vi "CTRE_Phoenix_CANdle_GetFaults.vi"(8 "error in":errorcluster, 11 "CTRE_CANdle_DeviceRef":T2) -> (0 "error out":errorcluster, 2 "Faults":T1, 3 "CTRE_CANdle_DeviceRef":T2)   [LabVIEW 2020]
doc: "Gets the current fault status of the CANdle."
uses:
  <vilib>/Rock Robotics/WPI/ThirdParty/Phoenix-LabVIEW/CANdle/Controls/CTRE_Phoenix_CANdle_DeviceRef.ctl
  <vilib>/Rock Robotics/WPI/ThirdParty/Phoenix-LabVIEW/CANdle/Controls/CTRE_Phoenix_CANdle_Faults.ctl
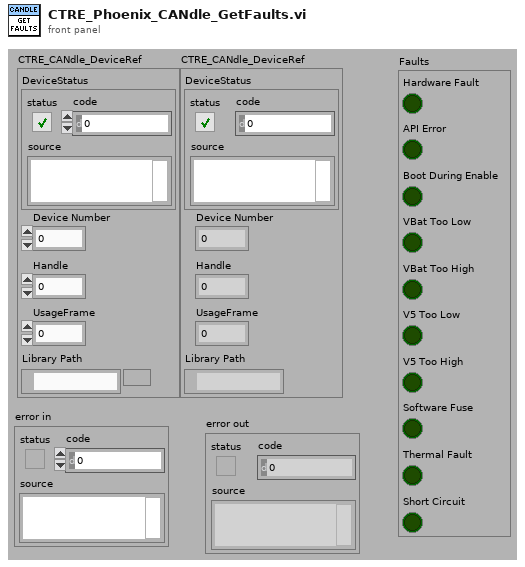
[diagram p1: front panel]
types:
  T1 = typedef "CTRE_Phoenix_CANdle_Faults.ctl" = cluster{"Hardware Fault":bool, "API Error":bool, "Boot During Enable":bool, "VBat Too Low":bool, "VBat Too High":bool, "V5 Too Low":bool, "V5 Too High":bool, "Software Fuse":bool, "Thermal Fault":bool, "Short Circuit":bool}
  T2 = typedef "CTRE_Phoenix_CANdle_DeviceRef.ctl" = cluster{"DeviceStatus":errorcluster, "Device Number":u8, "Handle":u64, "UsageFrame":u32, "Library Path":path}
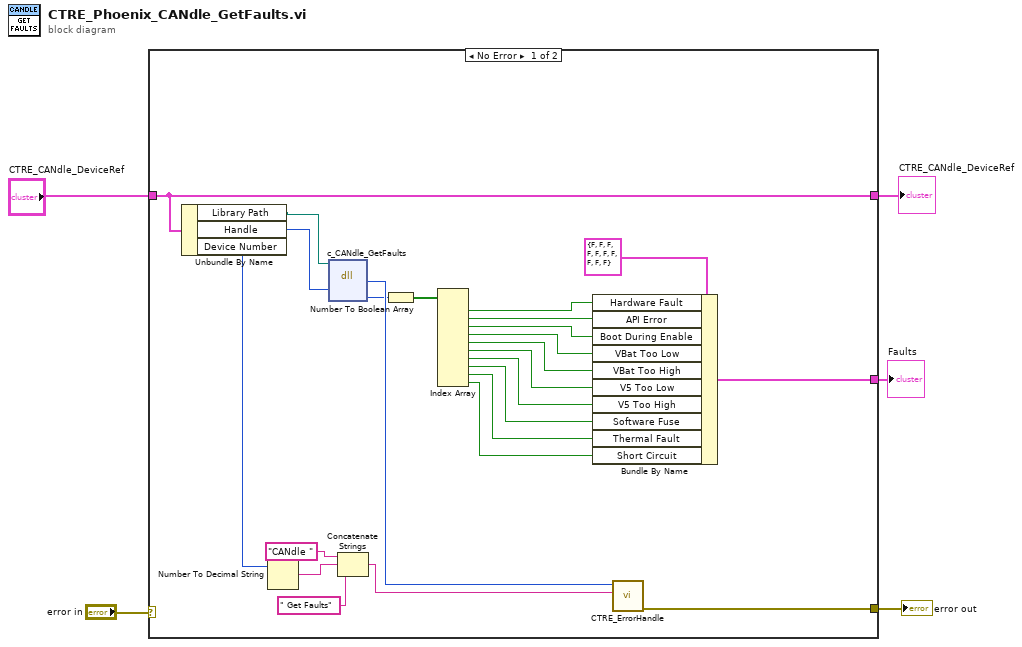
[diagram p0: block diagram]
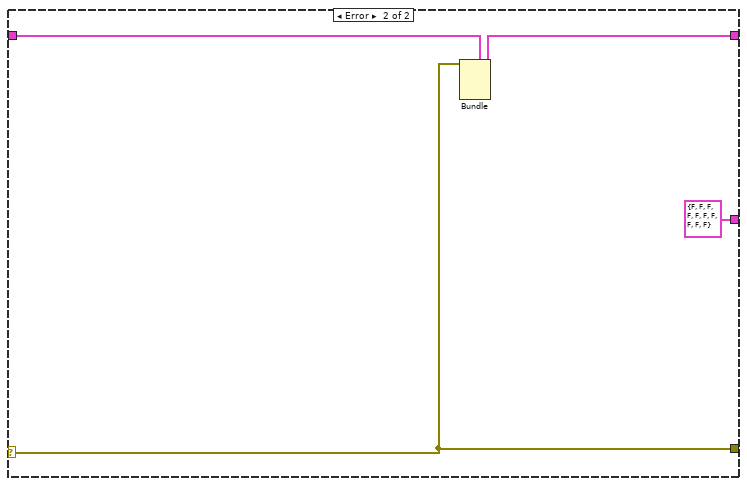
[diagram p2: hidden frame]
diagram:
  n1 = case shown="No Error" "error in" {
    selector: "error in" -> [_ w32]
    tunnel: "CTRE_CANdle_DeviceRef" -> [w19 w33]
    tunnel: [w29 w32] -> w5
    tunnel: [w19 w31] -> w2
    tunnel: [w6 T1 {"Hardware Fault"=FALSE, "API Error"=FALSE, "Boot During Enable"=FALSE, "VBat Too Low"=FALSE, "VBat Too High"=FALSE, "V5 Too Low"=FALSE, "V5 Too High"=FALSE, "Software Fuse"=FALSE, "Thermal Fault"=FALSE, "Short Circuit"=FALSE}] -> w1
    frame No Error {
      n2 = Unbundle By Name(w19) -> ("Library Path"=w18:path, "Handle"=w17:u64, "Device Number"=w16:u8)
      n3 = Number To Decimal String(number=w16) -> (decimal integer string=w21:string)  [unwired: 1 in]
      n4 = dll-call lib="?" fn="c_CANdle_GetFaults"(path in=w18, "handle"=w17) -> ("ErrorCode"=w28:i32, "faults"=w27:i32)  [unwired: 4 in, 2 out]
      n5 = Concatenate Strings("CANdle " ("string"), w21, " Get Faults" ("string")) -> (w15:string)
      n6 = Number To Boolean Array(number=w27) -> (Boolean array=w26:bool[])
      n7 = Index Array(array=w26) -> (element #1=w25:bool, element #2=w24:bool, element #3=w23:bool, element #4=w22:bool, element #5=w12:bool, element #6=w11:bool, element #7=w10:bool, element #8=w9:bool, element #9=w8:bool, element #10=w7:bool)  [unwired: 10 in]
      n8 = Bundle By Name(cluster=T1 {"Hardware Fault"=FALSE, "API Error"=FALSE, "Boot During Enable"=FALSE, "VBat Too Low"=FALSE, "VBat Too High"=FALSE, "V5 Too Low"=FALSE, "V5 Too High"=FALSE, "Software Fuse"=FALSE, "Thermal Fault"=FALSE, "Short Circuit"=FALSE}, "Hardware Fault"=w25, "API Error"=w24, "Boot During Enable"=w23, "VBat Too Low"=w22, "VBat Too High"=w12, "V5 Too Low"=w11, "V5 Too High"=w10, "Software Fuse"=w9, "Thermal Fault"=w8, "Short Circuit"=w7) -> (w6:T1)
      n9 = call <vilib>:"CTRE_ErrorHandle.vi"("origin"=w15, "code"=w28) -> ("error out"=w29:errorcluster)  [unwired: 9 in]
    }
    frame Error {
      n10 = Bundle(cluster=w33, "DeviceStatus"=w32) -> (w31:T2)  [unwired: 4 in]
    }
  }
  "error out" <- w5
  "CTRE_CANdle_DeviceRef" <- w2
  "Faults" <- w1
